vi "PV Software Current State.vi"(11 "HEX Data (U8)":u8) -> (3 "Current State":string)   [LabVIEW 2023]
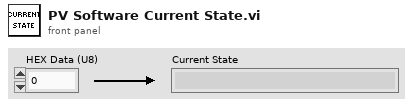
[diagram p1: front panel]
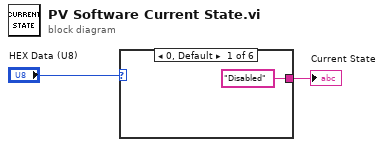
[diagram p0: block diagram]
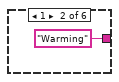
[diagram p2: hidden frame]
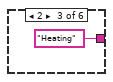
[diagram p3: hidden frame]
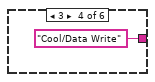
[diagram p4: hidden frame]
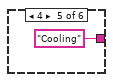
[diagram p5: hidden frame]
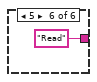
[diagram p6: hidden frame]
diagram:
  n1 = case shown="0, Default" "HEX Data (U8)" {
    tunnel: ["Disabled" "Warming" "Heating" "Cool/Data Write" "Cooling" "Read"] -> w1
    frame 0, Default {
    }
    frame 1 {
    }
    frame 2 {
    }
    frame 3 {
    }
    frame 4 {
    }
    frame 5 {
    }
  }
  "Current State" <- w1
